vi "ProgG_007_MG.vi"() -> ()   [LabVIEW 2021]
panel:
  out "Czas obliczeń [s]":dbl=0.101
  in  "Różnica ciągu arytmetycznego":dbl=6.0
  in  "Pierwszy wyraz":dbl=5.0
  in  "Któy wyraz ciągu obliczyć?\nN":i64=99999999
  out "Obliczony wyraz ciągu":i64=599999993
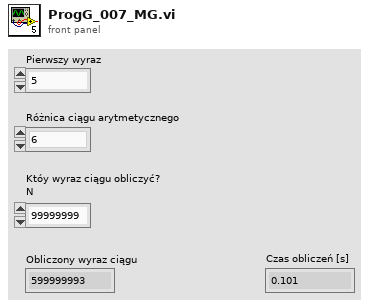
[diagram p1: front panel]
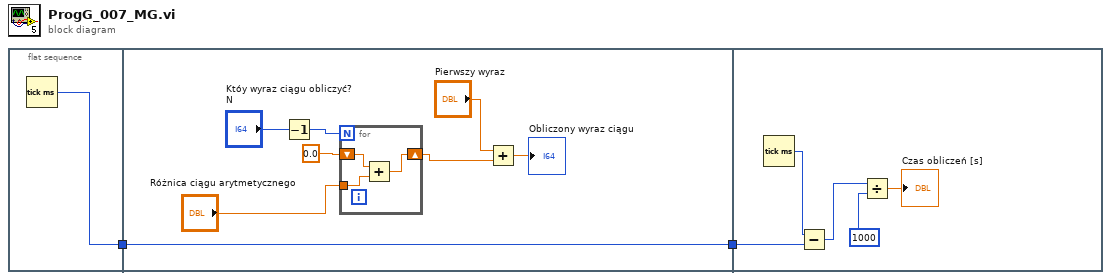
[diagram p0: block diagram]
diagram:
  n1 = flat-sequence {
    tunnel: [w3] -> w2
    tunnel: [w11] -> w1
    tunnel: w2 -> [w11]
    tunnel: w1 -> [w19]
    frame #0 {
      n2 = Tick Count (ms)() -> (millisecond timer value=w3:u32)
    }
    frame #1 {
      n3 = Decrement(x="Któy wyraz ciągu obliczyć?\nN") -> (x-1=w7:i64)
      n4 = for {
        N: w7 -> [_]
        tunnel: "Różnica ciągu arytmetycznego" -> [w14]
        shift-right: [w12] -> w4
        shift-left: 0.0 ("x") -> [w13]
        n5 = Add(x=w13, y=w14) -> (x+y=w12:dbl)
      }
      n6 = Add(x="Pierwszy wyraz", y=w4) -> (x+y=→"Obliczony wyraz ciągu":dbl)
    }
    frame #2 {
      n7 = Tick Count (ms)() -> (millisecond timer value=w18:u32)
      n8 = Subtract(x=w18, y=w19) -> (x-y=w16:u32)
      n9 = Divide(x=w16, y=u32 1000) -> (x/y=→"Czas obliczeń [s]":dbl)
    }
  }
